vi "TCPROSSubscriberInit.vi"(2 "topic":string, 3 "callerID":string) -> (0 "Success?":bool, 1 "TCP ROS Reply":string)   [LabVIEW 2010]
uses:
  <userlib>/ROSforLV_0.1/ROS/MessageBuilding/Primitives/subs/stringArray.vi
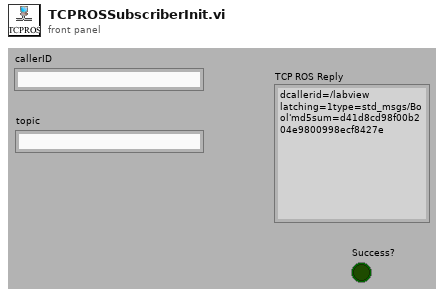
[diagram p1: front panel]
types:
  T1 = typedef "_ROSControl.ctl" = cluster{"topic port":u16, "Node":string, "topic":string, "type":string, "node port":u32, "error ":errorcluster, "Direction":T2, "APIs":string[]}
  T2 = typedef "_ROSDirection.ctl" = enum16{"Node", "Publisher", "Subscriber", "Service Client"}
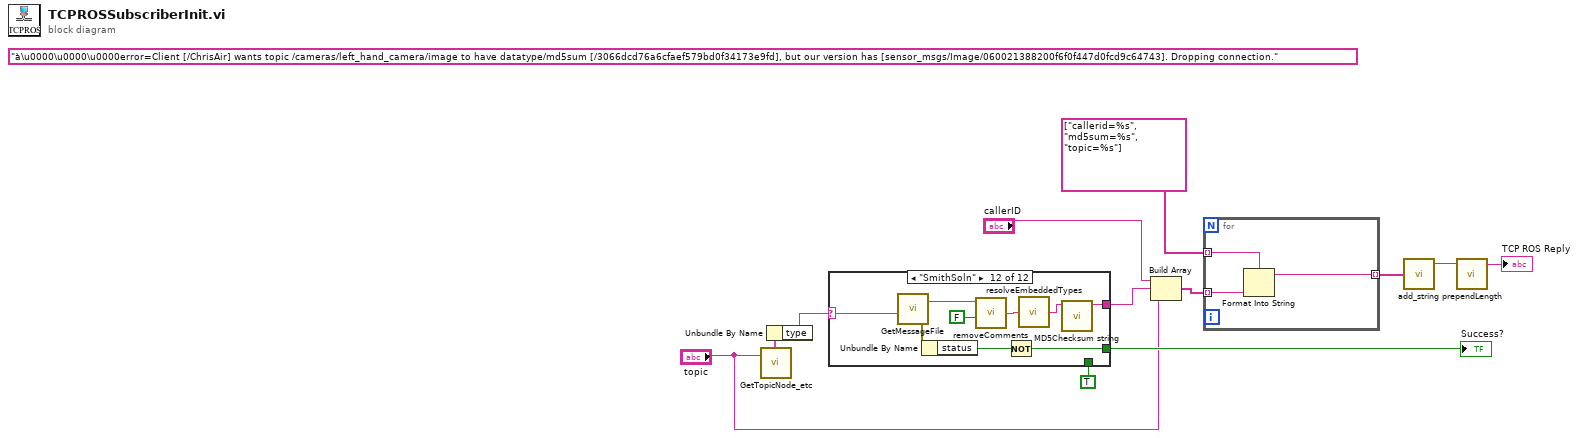
[diagram p0: block diagram]
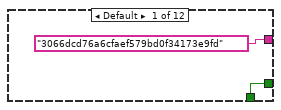
[diagram p2: hidden frame]
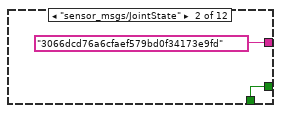
[diagram p3: hidden frame]
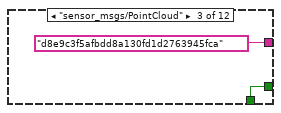
[diagram p4: hidden frame]
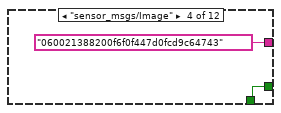
[diagram p5: hidden frame]
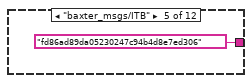
[diagram p6: hidden frame]
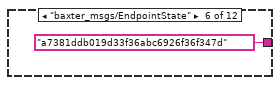
[diagram p7: hidden frame]
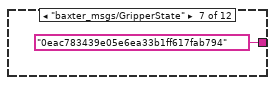
[diagram p8: hidden frame]
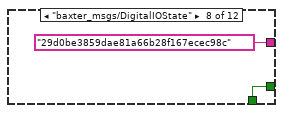
[diagram p9: hidden frame]
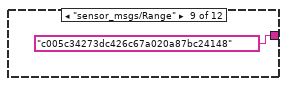
[diagram p10: hidden frame]
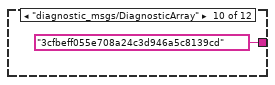
[diagram p11: hidden frame]
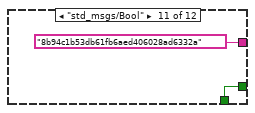
[diagram p12: hidden frame]
diagram:
  (unwired) "à\u0000\u0000\u0000error=Client [/ChrisAir] wants topic /cameras/left_hand_camera/image to have datatype/md5sum [/3066dcd76a6cfaef579bd0f34173e9fd], but our version has [sensor_msgs/Image/060021388200f6f0f447d0fcd9c64743]. Dropping connection." ("Second")
  n1 = call <userlib>:"GetTopicNode_etc.vi"("topic"="topic") -> ("Baxter"=w8:T1)  [unwired: 2 in]
  n2 = Unbundle By Name(w8) -> ("type"=w7:string)
  n3 = case shown="\"SmithSoln\"" w7 {
    selector: w7 -> [_ _ _ _ _ _ _ _ _ _ _ w34]
    tunnel: ["3066dcd76a6cfaef579bd0f34173e9fd" "3066dcd76a6cfaef579bd0f34173e9fd" "d8e9c3f5afbdd8a130fd1d2763945fca" "060021388200f6f0f447d0fcd9c64743" ("MD5 Sum") "fd86ad89da05230247c94b4d8e7ed306" ("MD5 Sum") "a7381ddb019d33f36abc6926f36f347d" ("MD5 Sum") "0eac783439e05e6ea33b1ff617fab794" ("MD5 Sum") "29d0be3859dae81a66b28f167ecec98c" ("MD5 Sum") "c005c34273dc426c67a020a87bc24148" ("Second") "3cfbeff055e708a24c3d946a5c8139cd" ("MD5 Sum") "8b94c1b53db61fb6aed406028ad6332a" ("MD5 Sum") w30] -> w10
    tunnel: [w14 w15 w17 w19 _ _ _ w24 _ _ w28 w32] -> w9
    tunnel: TRUE ("status") -> [w14 w15 w17 w19 _ _ _ w24 _ _ w28 _]
    frame Default {
    }
    frame "sensor_msgs/JointState" {
    }
    frame "sensor_msgs/PointCloud" {
    }
    frame "sensor_msgs/Image" {
    }
    frame "baxter_msgs/ITB" {
    }
    frame "baxter_msgs/EndpointState" {
    }
    frame "baxter_msgs/GripperState" {
    }
    frame "baxter_msgs/DigitalIOState" {
    }
    frame "sensor_msgs/Range" {
    }
    frame "diagnostic_msgs/DiagnosticArray" {
    }
    frame "std_msgs/Bool" {
    }
    frame "SmithSoln" {
      n4 = call <userlib>:"GetMessageFile.vi"("type"=w34) -> ("error out"=w35:errorcluster, "File"=w36:string)  [unwired: 1 in]
      n5 = Unbundle By Name(w35) -> ("status"=w33:bool)
      n6 = call <userlib>:"removeComments.vi"("Trim Whitespace? (F)"=FALSE ("Trim Whitespace?"), "String"=w36) -> ("Body"=w38:string)  [unwired: 2 in, 2 out]
      n7 = Not(x=w33) -> (.not. x?=w32:bool)
      n8 = call <userlib>:"resolveEmbeddedTypes.vi"("Message Definition"=w38) -> ("Md5 Text"=w31:string)
      n9 = call <vilib>:"MD5Checksum string.vi"("Message String"=w31) -> ("MD5 message-digest"=w30:string)  [unwired: 10 in]
    }
  }
  "Success?" <- w9
  n10 = Build Array("callerID", w10, "topic") -> (w11:string[])
  n11 = for {
    tunnel: w11 -> [w40] mode=indexing
    tunnel: string[] ["callerid=%s", "md5sum=%s", "topic=%s"] -> [w41] mode=indexing
    tunnel: [w39] -> w3 mode=indexing
    n12 = Format Into String(format string=w41, w40) -> (resulting string=w39:string)  [unwired: 2 in, 1 out]
  }
  n13 = call-poly <userlib>:"add_string.vi"("Array"=w3) -> ("msg out"=w2:string)  [unwired: 4 in]
  n14 = call <userlib>:"prependLength.vi"("msg in"=w2) -> ("msg out"=→"TCP ROS Reply":string)  [unwired: 4 in]
